vi "DMM6500_Create All Message Queues.vi"(8 "error in (no error)":errorcluster, 11 "This VI":refnum<vi>) -> (0 "error out":errorcluster, 3 "Message Queues out":T1)   [LabVIEW 2024, in "DMM6500.lvlib" / "DMM6500 Message Queue.lvlib"]
doc: "This VI creates and initializes all the message queues for your application. If your application requires more than one message queue, right-click the \"Message Queues\" constant above and select Open Type Def. Add the new Message Queue(s) to the type definition, then initialize them in this VI."
uses:
  DMM6500 Message Queue.lvlib
  DMM6500_All Message Queues.ctl
  DMM6500_Enqueue Message (Single).vi
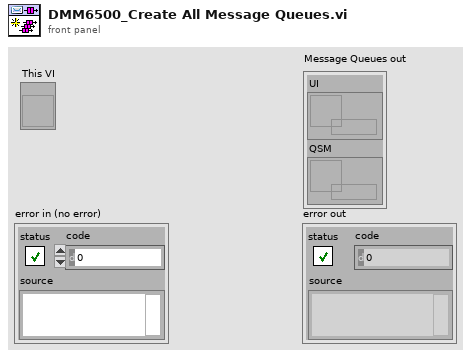
[diagram p1: front panel]
types:
  T1 = typedef "DMM6500.lvlib/DMM6500 Message Queue.lvlib/DMM6500_All Message Queues.ctl" = cluster{"UI":refnum<queue>, "QSM":refnum<queue>}
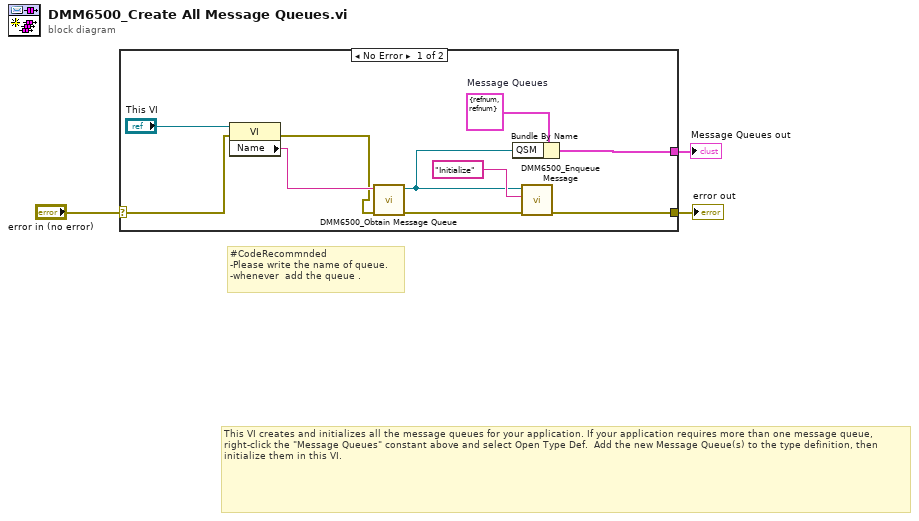
[diagram p0: block diagram]
diagram:
  # "#CodeRecommnded\n-Please write the name of queue.\n-whenever  add the queue ."
  # "This VI creates and initializes all the message queues for your application. If your application requires more than one message queue, right-click the \"Message Queues\" constant above and select Open Type Def.  Add the new Message Queue(s) to the type definition, then initialize them in this VI."
  n1 = case shown="No Error" "error in (no error)" {
    selector: "error in (no error)" -> [w5 w14]
    tunnel: [w13 w14] -> w3
    tunnel: [w11 _] -> w2
    frame No Error {
      w12 = T1 {"UI"=refnum, "QSM"=refnum}  # Message Queues
      n2 = property class="VI"(reference="This VI", error in=w5) -> (error out=w4:errorcluster, "Name"=w7:string)  [unwired: 1 out]
      n3 = call "DMM6500_Obtain Message Queue.vi"("error in (no error)"=w4, "Queue Name"=w7) -> ("error out"=w10:errorcluster, "Message Queue"=w8:refnum<queue>)  [unwired: 8 in]
      n4 = Bundle By Name(cluster=w12, "QSM"=w8) -> (w11:T1)
      n5 = call-poly "DMM6500_Enqueue Message.vi"("error in (no error)"=w10, "Message"="Initialize", "Message Queue"=w8) -> ("error out"=w13:errorcluster)  [unwired: 7 in, 1 out]
    }
    frame Error {
    }
  }
  "Message Queues out" <- w2
  "error out" <- w3
